vi "Meta.vi"() -> ()   [LabVIEW 2019]
panel:
  in  "Tab Control":enum32{"ReFORM", "Iterate Main"}(tab)=enum."Iterate Main"
  in  "FORM cells":string="731\n15843\n21211\n21899\n25059\n29643\n29803\n31979\n32243\n32491\n38643\n39139\n42739\n43507\n43755\n46315\n47779\n48043\n48867\n49115\n49395\n49643\n55499\n56715\n57307\n58267\n58291\n60251\n61387\n62411\n62947\n63635\n64467"
  out "FORM array":u16[](array[numeric])=[731, 15843, 21211, 21899, 25059, 29643, 29803, 31979, 32243, 32491, 38643, 39139, 42739, 43507, 43755, 46315, 47779, 48043, 48867, 49115, 49395, 49643, 55499, 56715, 57307, 58267, 58291, 60251, 61387, 62411, 62947, 63635, 64467]
  in  "Iterations":i32=5
  in  "Initial address":u16
  in  "Final address":u16=65535
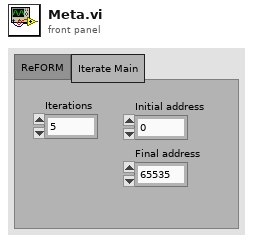
[diagram p1: front panel]
types:
  T1 = enum32{"FORM", "SET", "RESET", "READ", "Target", "CB (W)", "CB (R)"}
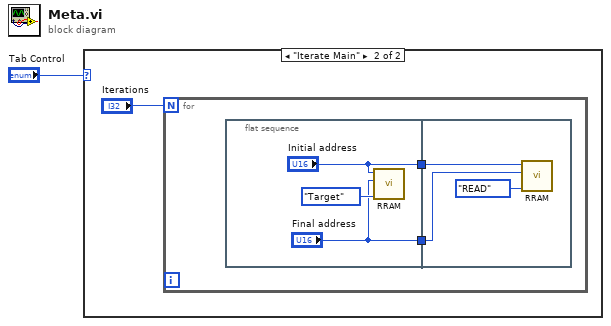
[diagram p0: block diagram]
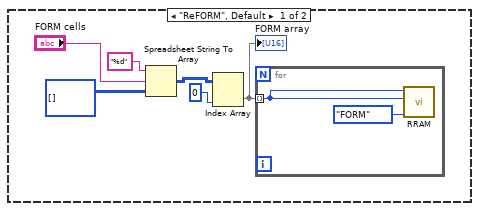
[diagram p2: hidden frame]
diagram:
  n1 = case shown="\"Iterate Main\"" "Tab Control" {
    frame "ReFORM", Default {
      n2 = Spreadsheet String To Array(format string="%d", spreadsheet string="FORM cells", array type (2D Dbl)=u16[][] []) -> (array=w4:u16[][])  [unwired: 1 in]
      n3 = Index Array(array=w4, index (col)=0 ("disabled index (col)")) -> (element=w2:u16[])  [unwired: 1 in]
      "FORM array" <- w2
      n4 = for {
        tunnel: w2 -> [w9] mode=indexing
        n5 = call "RRAM.vi"("Mode"=T1."FORM", "Final address"=w9, "Initial address"=w9) -> ()  [unwired: 9 in]
      }
    }
    frame "Iterate Main" {
      n6 = for {
        N: "Iterations" -> [_]
        n7 = flat-sequence {
          tunnel: ["Final address"] -> w12
          tunnel: ["Initial address"] -> w11
          tunnel: w12 -> [w17]
          tunnel: w11 -> [w16]
          frame #0 {
            n8 = call "RRAM.vi"("Mode"=T1."Target", "Final address"="Final address", "Initial address"="Initial address") -> ()  [unwired: 9 in]
          }
          frame #1 {
            n9 = call "RRAM.vi"("Mode"=T1."READ", "Final address"=w17, "Initial address"=w16) -> ()  [unwired: 9 in]
          }
        }
      }
    }
  }
